vi "Set I32.vi"(8 "error in (no error)":errorcluster, 10 "Numeric":i32, 11 "JSON Scalar in":refnum<class "JSON Scalar.lvclass">) -> (0 "error out":errorcluster, 3 "JSON Scalar out":refnum<class "JSON Scalar.lvclass">)   [LabVIEW 2011, in "JSON Scalar.lvclass"]
doc: "Stores a <b>Numeric</b> as a <b>JSON Scalar</b>.\n\nCopyright 2012 James David Powell, Shaun Rumbell and Ton Plomp\nMore information on http://lavag.org/topic/16217-cr-json-labview"
uses:
  JSON Scalar.lvclass
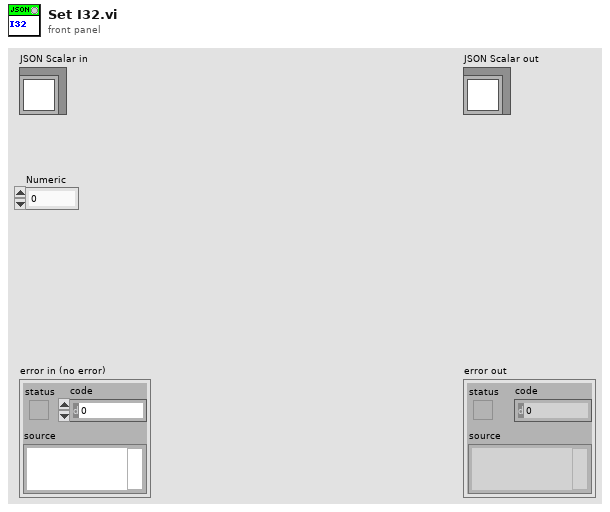
[diagram p1: front panel]
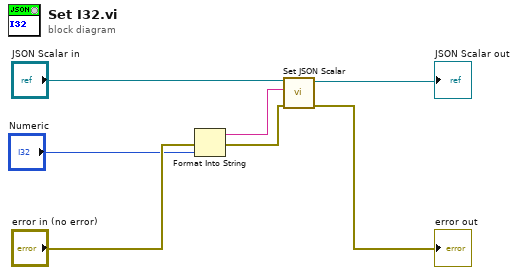
[diagram p0: block diagram]
diagram:
  n1 = Format Into String(error in="error in (no error)", "Numeric") -> (resulting string=w2:string, error out=w1:errorcluster)  [unwired: 2 in]
  n2 = call "Set JSON Scalar.vi"("error in (no error)"=w1, "LabVIEW Text"=w2, "JSON Scalar in"="JSON Scalar in") -> ("error out"=→"error out":errorcluster, "JSON Scalar out"=→"JSON Scalar out":refnum<class "JSON Scalar.lvclass">)  [unwired: 7 in]
